vi "Proceso de moneda.vi"(8 "error in (no error)":errorcluster, 10 "Coins":cluster{"$1":bool, "$2":bool, "$5":bool}, 11 "MXN ACTOR in":refnum<class "MXN ACTOR.lvclass">) -> (0 "error out":errorcluster, 3 "MXN ACTOR out":refnum<class "MXN ACTOR.lvclass">)   [LabVIEW 2019, in "MXN ACTOR.lvlib" / "MXN ACTOR.lvclass"]
uses:
  MXN ACTOR.lvclass
  C:/Program Files (x86)/National Instruments/LabVIEW 2019/vi.lib/ActorFramework/Actor/Actor.lvclass
  <vilib>/ActorFramework/Actor/Actor.lvclass/Actor.ctl
  MXN ACTOR.lvclass/MXN ACTOR.ctl
  UI Actor Messages/Credit update1 Msg/Credit update1 Msg.lvclass/Credit update1 Msg.ctl
  <vilib>/ActorFramework/Message Enqueuer/Message Enqueuer.lvclass/Message Enqueuer.ctl
  <vilib>/ActorFramework/Message Enqueuer/Enqueue.vi
  UI Actor Messages/Credit update1 Msg/Credit update1 Msg.lvclass
  C:/Program Files (x86)/National Instruments/LabVIEW 2019/vi.lib/ActorFramework/Message/Message.lvclass
  <vilib>/ActorFramework/Message Priority Queue/Priority Enqueue.vi
  <vilib>/ActorFramework/Actor/Actor.lvclass
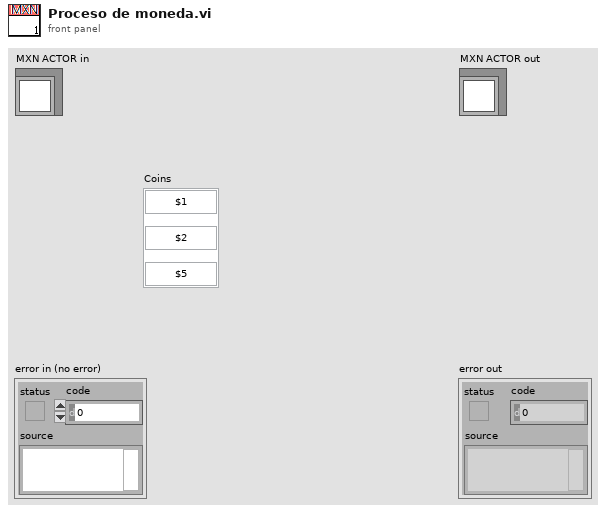
[diagram p1: front panel]
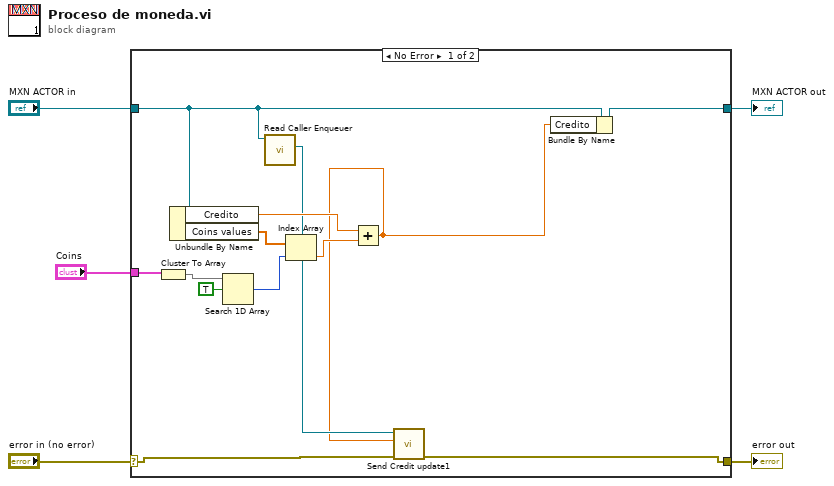
[diagram p0: block diagram]
diagram:
  n1 = case shown="No Error" "error in (no error)" {
    selector: "error in (no error)" -> [w7 w20]
    tunnel: [w6 w20] -> w4
    tunnel: [w11 w19] -> w2
    tunnel: "MXN ACTOR in" -> [w10 w19]
    tunnel: "Coins" -> [w18 _]
    frame No Error {
      n2 = Cluster To Array(cluster=w18) -> (array=w17:bool[])
      n3 = Unbundle By Name(w10) -> ("Credito"=w12:dbl, "Coins values"=w15:dbl[])
      n4 = Search 1D Array(1D array=w17, element=TRUE) -> (index of element=w14:i32)  [unwired: 1 in]
      n5 = call <vilib>:"Read Caller Enqueuer.vi"("Actor"=w10) -> ("Caller Enqueuer"=w9:refnum<class "Message Enqueuer.lvclass">)  [unwired: 10 in]
      n6 = Index Array(array=w15, index=w14) -> (element=w13:dbl)
      n7 = Add(x=w12, y=w13) -> (x+y=w8:dbl)
      n8 = call "Send Credit update1.vi"("error in (no error)"=w7, "Credit"=w8, "Message Enqueuer"=w9) -> ("error out"=w6:errorcluster)  [unwired: 7 in, 1 out]
      n9 = Bundle By Name(cluster=w10, "Credito"=w8) -> (w11:refnum<class "MXN ACTOR.lvclass">)
    }
    frame Error {
    }
  }
  "error out" <- w4
  "MXN ACTOR out" <- w2
